vi "verify errors.vi"(8 "error in (no error)":errorcluster, 11 "Channel in":refnum<class "SPARC4_Channel.lvclass">) -> (0 "error out":errorcluster, 2 "error":bool, 3 "Channel out":refnum<class "SPARC4_Channel.lvclass">)   [LabVIEW 2018, in "SPARC4_Channel.lvclass"]
uses:
  SPARC4_Channel.lvclass
  SPARC4_Channel.lvclass/SPARC4_Channel.ctl
  Sim_CCD/Sim_CCD.lvclass/Sim_CCD.ctl
  Sim_CCD/Sim_CCD.lvclass
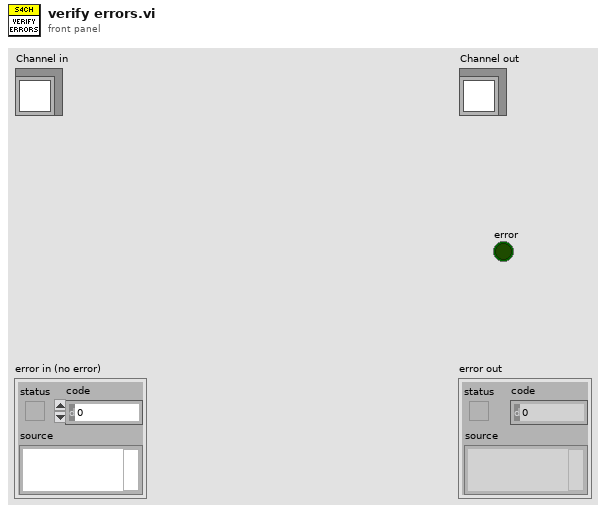
[diagram p1: front panel]
types:
  T1 = cluster{"#CYCLES":errorcluster, "SUFFIX":errorcluster}
  T2 = cluster{"#SEQS":errorcluster, "WAVEPLATE_POS":errorcluster}
  T3 = cluster{"State Machine.lvclass":refnum<class "State Machine.lvclass">, "RxTx.lvclass":refnum<class "RxTx.lvclass">, "Save_Header_RxTx.lvclass":refnum<class "RxTx.lvclass">, "Status SM.lvclass":refnum<class "State Machine.lvclass">, "Status RxTx.lvclass":refnum<class "RxTx.lvclass">, "servers array":refnum<class "Server.lvclass">[], "Events log file.lvclass":refnum<class "Log File.lvclass">, "Errors log file.lvclass":refnum<class "Log File.lvclass">, "Keywords log file.lvclass":refnum<class "Log File.lvclass">, "Sim_CCD.lvclass":refnum<class "Sim_CCD.lvclass">}
  T4 = cluster{"EXPTIME":errorcluster, "#FRAMES":errorcluster}
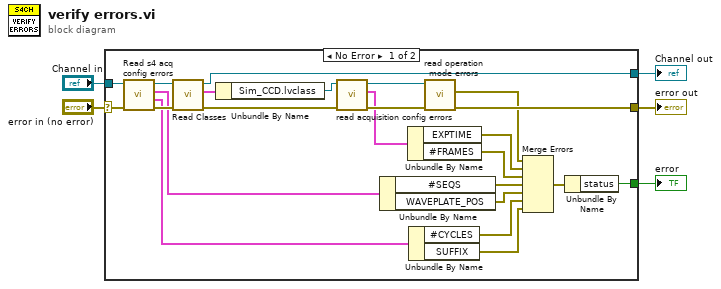
[diagram p0: block diagram]
diagram:
  n1 = case shown="No Error" "error in (no error)" {
    selector: "error in (no error)" -> [w11 w30]
    tunnel: [w26 w30] -> w4
    tunnel: [w16 w29] -> w2
    tunnel: "Channel in" -> [w13 w29]
    tunnel: [w24 _] -> w1
    frame No Error {
      n2 = call "Read s4 acq config errors.vi"("error in (no error)"=w11, "SPARC4_Channel in"=w13) -> ("error out"=w10:errorcluster, "acquisition config errors"=w8:T1, "s4 acq config errors"=w9:T2, "SPARC4_Channel out"=w12:refnum<class "SPARC4_Channel.lvclass">)  [unwired: 6 in]
      n3 = call-dynamic "Read Classes.vi"("error in (no error)"=w10, "Channel in"=w12) -> ("error out"=w17:errorcluster, "Classes"=w19:T3, "Channel out"=w16:refnum<class "SPARC4_Channel.lvclass">)  [unwired: 7 in]
      n4 = Unbundle By Name(w19) -> ("Sim_CCD.lvclass"=w18:refnum<class "Sim_CCD.lvclass">)
      n5 = call "read acquisition config errors.vi"("error in (no error)"=w17, "Simulated Camera in"=w18) -> ("error out"=w28:errorcluster, "acq config errors"=w22:T4, "Simulated Camera out"=w27:refnum<class "Sim_CCD.lvclass">)  [unwired: 7 in]
      n6 = Unbundle By Name(w9) -> ("#SEQS"=w15:errorcluster, "WAVEPLATE_POS"=w14:errorcluster)
      n7 = Unbundle By Name(w22) -> ("EXPTIME"=w21:errorcluster, "#FRAMES"=w20:errorcluster)
      n8 = Unbundle By Name(w8) -> ("#CYCLES"=w7:errorcluster, "SUFFIX"=w6:errorcluster)
      n9 = call "read operation mode errors.vi"("error in (no error)"=w28, "Simulated_CCD_Camera in"=w27) -> ("error out"=w26:errorcluster, "WRITE SETUP errors"=w23:errorcluster[])  [unwired: 7 in, 1 out]
      n10 = Merge Errors(w23, w21, w20, w15, w14, w7, w6) -> (w25:errorcluster)
      n11 = Unbundle By Name(w25) -> ("status"=w24:bool)
    }
    frame Error {
    }
  }
  "error out" <- w4
  "Channel out" <- w2
  "error" <- w1
